vi "Replace DAQ Controls.vi"(0 "VI in":refnum<vi>, 11 "error in (no error)":errorcluster) -> (4 "VI out":refnum<vi>, 15 "error out":errorcluster)   [LabVIEW 2021, in "Migrator.lvlib"]
uses:
  Migrator.lvlib
  <vilib>/Utility/traverseref.llb/TRef TravTarget.ctl
  <vilib>/Utility/traverseref.llb/VI Scripting - Traverse.lvlib
  Path Functions/Path Functions.lvlib
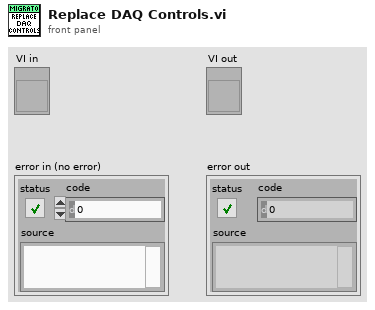
[diagram p1: front panel]
types:
  T1 = typedef "TRef TravTarget.ctl" = enum16{"FP", "BD", "Other"}
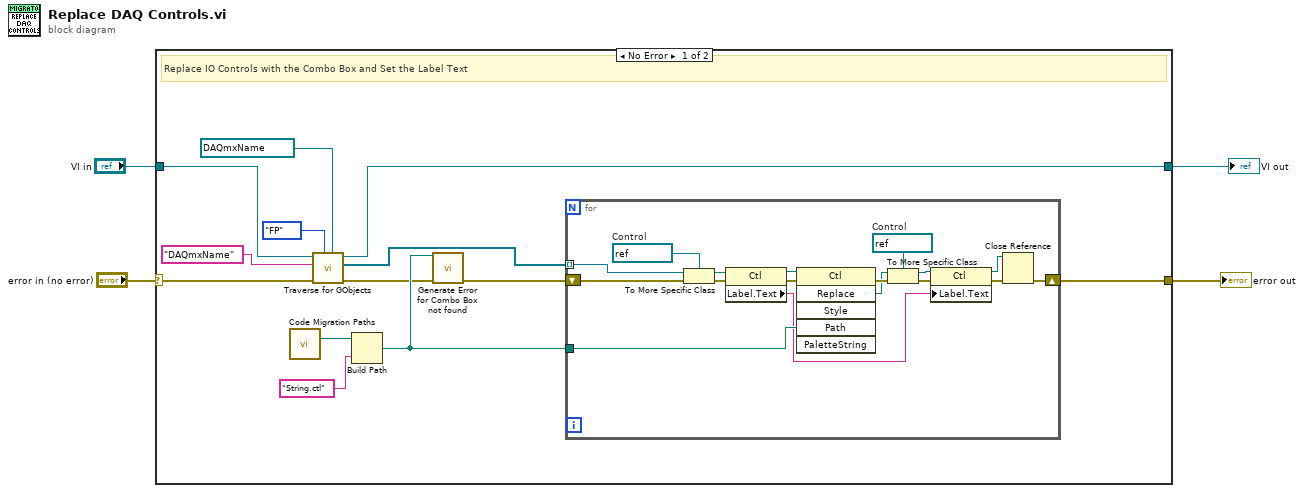
[diagram p0: block diagram]
diagram:
  n1 = case shown="No Error" "error in (no error)" {
    selector: "error in (no error)" -> [w14 w35]
    tunnel: [w6 w35] -> w4
    tunnel: [w16 w36] -> w3
    tunnel: "VI in" -> [w13 w36]
    frame No Error {
      # "Replace IO Controls with the Combo Box and Set the Label Text"
      n2 = call "Code Migration Paths.vi"() -> ("IO Controls"=w12:path)  [unwired: 7 in, 8 out]
      n3 = call <vilib>:"Traverse for GObjects.vi"("Other Refnum"=refnum<vi> refnum, "Traverse Target"=TRef_TravTarget."FP", "error in (no error)"=w14, "Class Name"="DAQmxName", "VI Refnum"=w13) -> ("error out"=w9:errorcluster, "References"=w7:refnum<vi>[], "dup VI Refnum"=w16:refnum<vi>)  [unwired: 3 in, 1 out]
      n4 = Build Path(base path=w12, name or relative path="String.ctl" ("string")) -> (appended path=w10:path)
      n5 = call "Generate Error for Combo Box not found.vi"("Template combox path"=w10, "error in (no error)"=w9) -> ("error out"=w8:errorcluster)  [unwired: 13 in]
      n6 = for {
        tunnel: w7 -> [w33] mode=indexing
        tunnel: w10 -> [w34]
        shift-right: [w18] -> w6
        shift-left: w8 -> [w32]
        w26 = refnum<vi> refnum  # Control
        w31 = refnum<vi> refnum  # Control
        n7 = To More Specific Class(target class=w31, reference=w33, error in=w32) -> (specific class reference=w30:refnum<vi>, error out=w28:errorcluster)
        n8 = property class="Ctl"(reference=w30, error in=w28) -> (reference out=w29:refnum<vi>, error out=w27:errorcluster, "Label.Text"=w21:string)
        n9 = invoke class="Ctl" method="Replace"(reference=w29, error in=w27, "Path"=w34) -> (error out=w25:errorcluster, "Replace"=w24:refnum<vi>)  [unwired: 3 in, 4 out]
        n10 = To More Specific Class(target class=w26, reference=w24, error in=w25) -> (specific class reference=w23:refnum<vi>, error out=w22:errorcluster)
        n11 = property class="Ctl"(reference=w23, error in=w22, "Label.Text"=w21) -> (reference out=w19:refnum<vi>, error out=w20:errorcluster)
        n12 = Close Reference(reference=w19, error in (no error)=w20) -> (error out=w18:errorcluster)
      }
    }
    frame Error {
    }
  }
  "error out" <- w4
  "VI out" <- w3
